vi "Data_get.vi"() -> ()   [LabVIEW 2009]
uses:
  <vilib>/Analysis/2dsp.llb/Real FFT.vi
  <vilib>/Analysis/NI_AALPro.lvlib
panel:
  in  "Auto":bool caption="Autosave"
  in  "FFT every#":u32=1 min=1 max=1000 step=1
  in  "#steps":u32=1 min=1 step=1
  in  "f step (MHz)":dbl=0.0003 min=0.00025 max=67.0 step=1e-06 format="%#.12f"
  in  "ps/point":T1(ring)
  in  "ns/div":T2(ring)
  out "Current sweep":u32=1 min=1 max=1000 step=1
  in  "Ext":string="ccd"
  out "f cur. (MHz)":string
  in  "Name":string="trace"
  in  "Folder":path
  in  "#Sweeps":u32=1 min=1 max=1000 step=1
  in  "Ampl. (dBm)":dbl min=-135.0 max=30.0 step=0.5 format="%#_8g"
  in  "f start (MHz)":dbl=0.0003 min=0.00025 max=67.0 step=1e-06 format="%#.12f"
  in  "Start":bool
  in  "Quit":bool
  in  "E8257D VISA Port":refnum<visa-resource-name>="GPIB0::1::INSTR"
  out "read time (ms)":u32
  out "#points":u32
  out "Busy":bool
  in  "Repetition rate (Hz)":ext=2.5
  in  "Chirp start (MHz)":ext=2.5
  in  "Filter up to (MHz)":ext=2.5
  in  "Amount of averagings":u32=10
  out "Data":dbl[](array[numeric])
  out "XY Graph 5":cluster{ext[], dbl[]}(graph)
  out "FFT (Im)":dbl[](array[numeric])
  out "FFT (Re)":dbl[](array[numeric])
  out "Final array":ext[][](array[numeric])
  out "size(s)":i32
  out "Oscilloscope Data":dbl[](array[numeric])
  in  "Channel Number":u16=1
  out "Oscilloscope graph":dbl[](graph)
  in  "Stop":bool
  in  "TDS VISA Port":refnum<visa-resource-name>="GPIB0::1::INSTR"
  # "TDS6000"
  # "E8257D"
  # "File Storage"
  # "Control"
  # "Spectrum data"
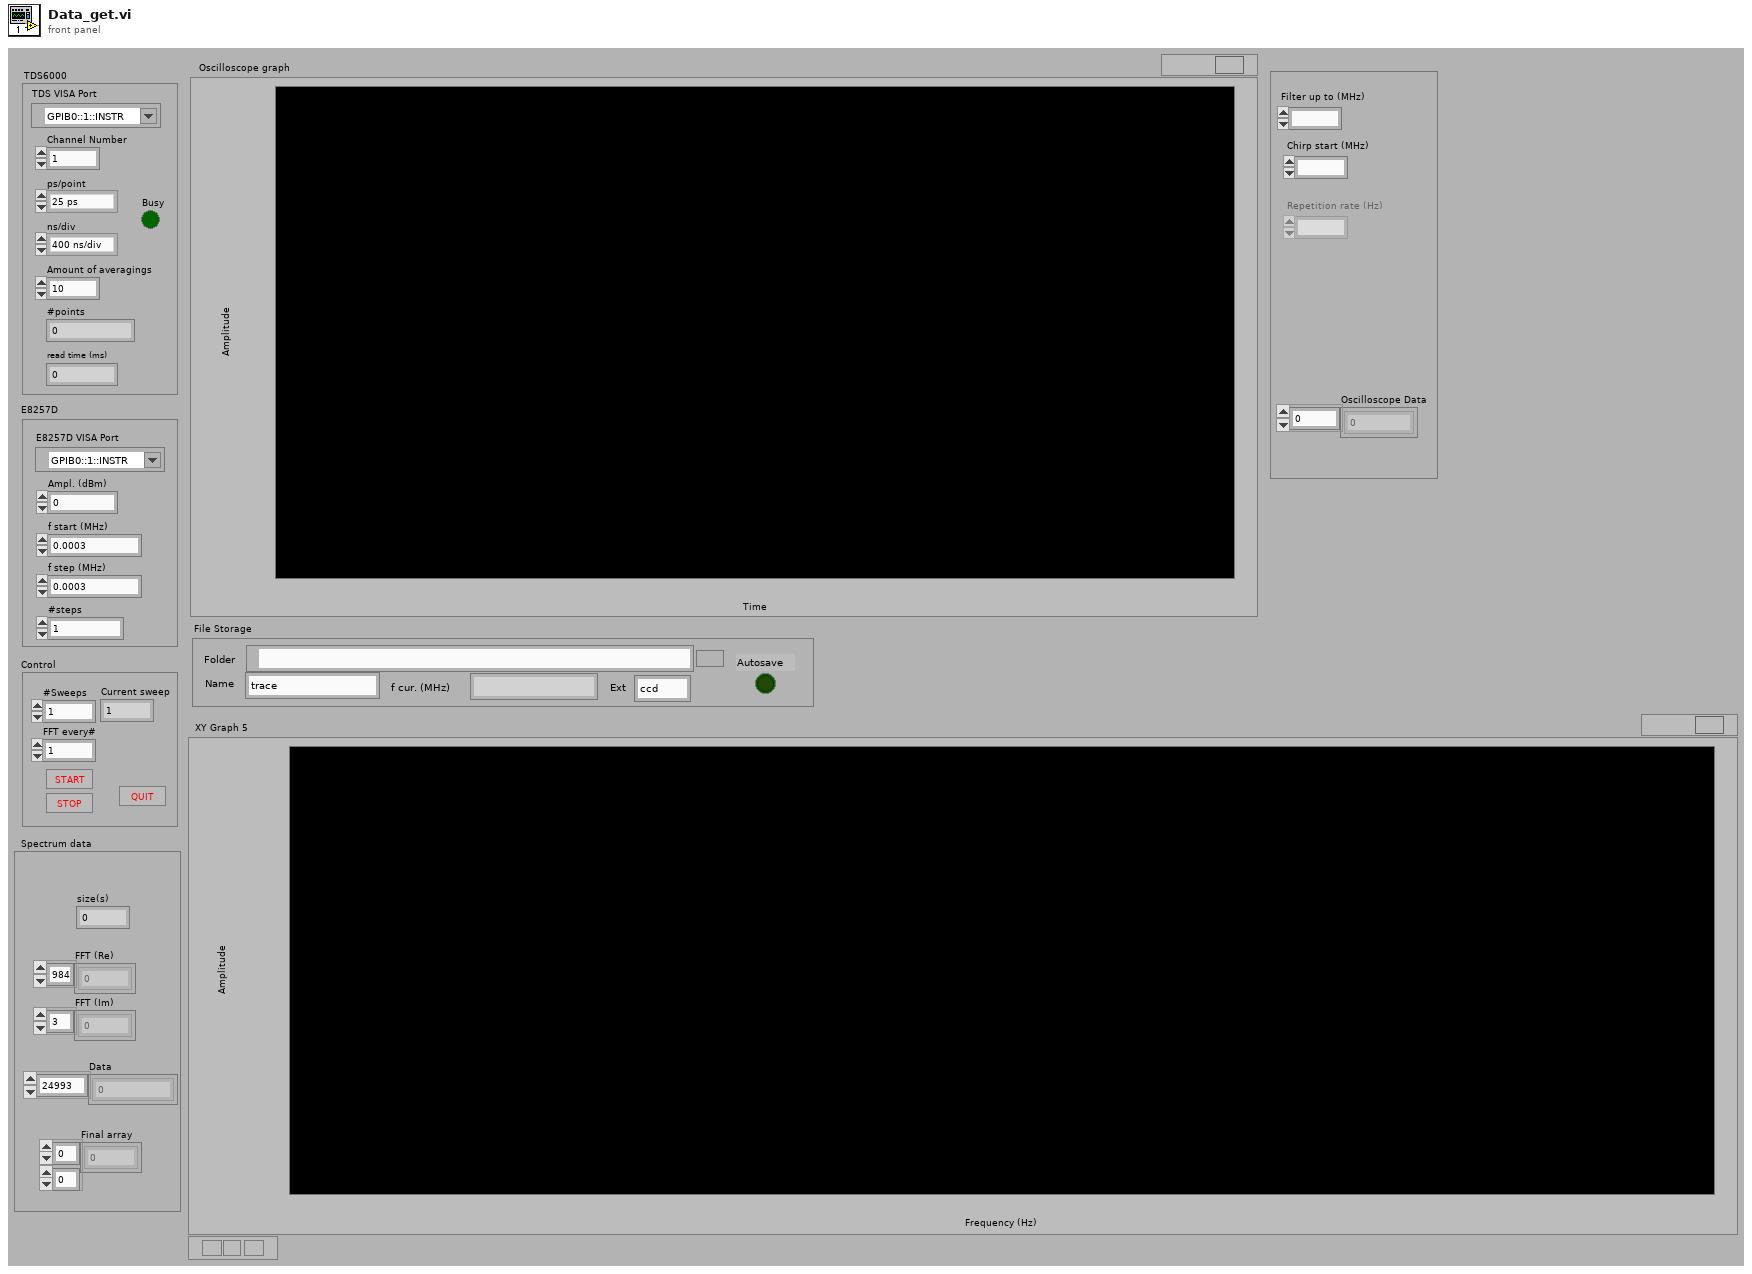
[diagram p1: front panel]
types:
  T1 = enum16{"25 ps", "50 ps", "100 ps", "200 ps", "400 ps", "800 ps", "2 ns"}
  T2 = enum16{"400 ns/div", "1 us/div", "2 us/div", "4 us/div", "10 us/div", "20 us/div"}
  T3 = enum16{"open", "replace", "create", "open or create", "replace or create", "replace or create with confirmation"}
  T4 = cluster{"Folder":path, "Name":string, "Ext":string}
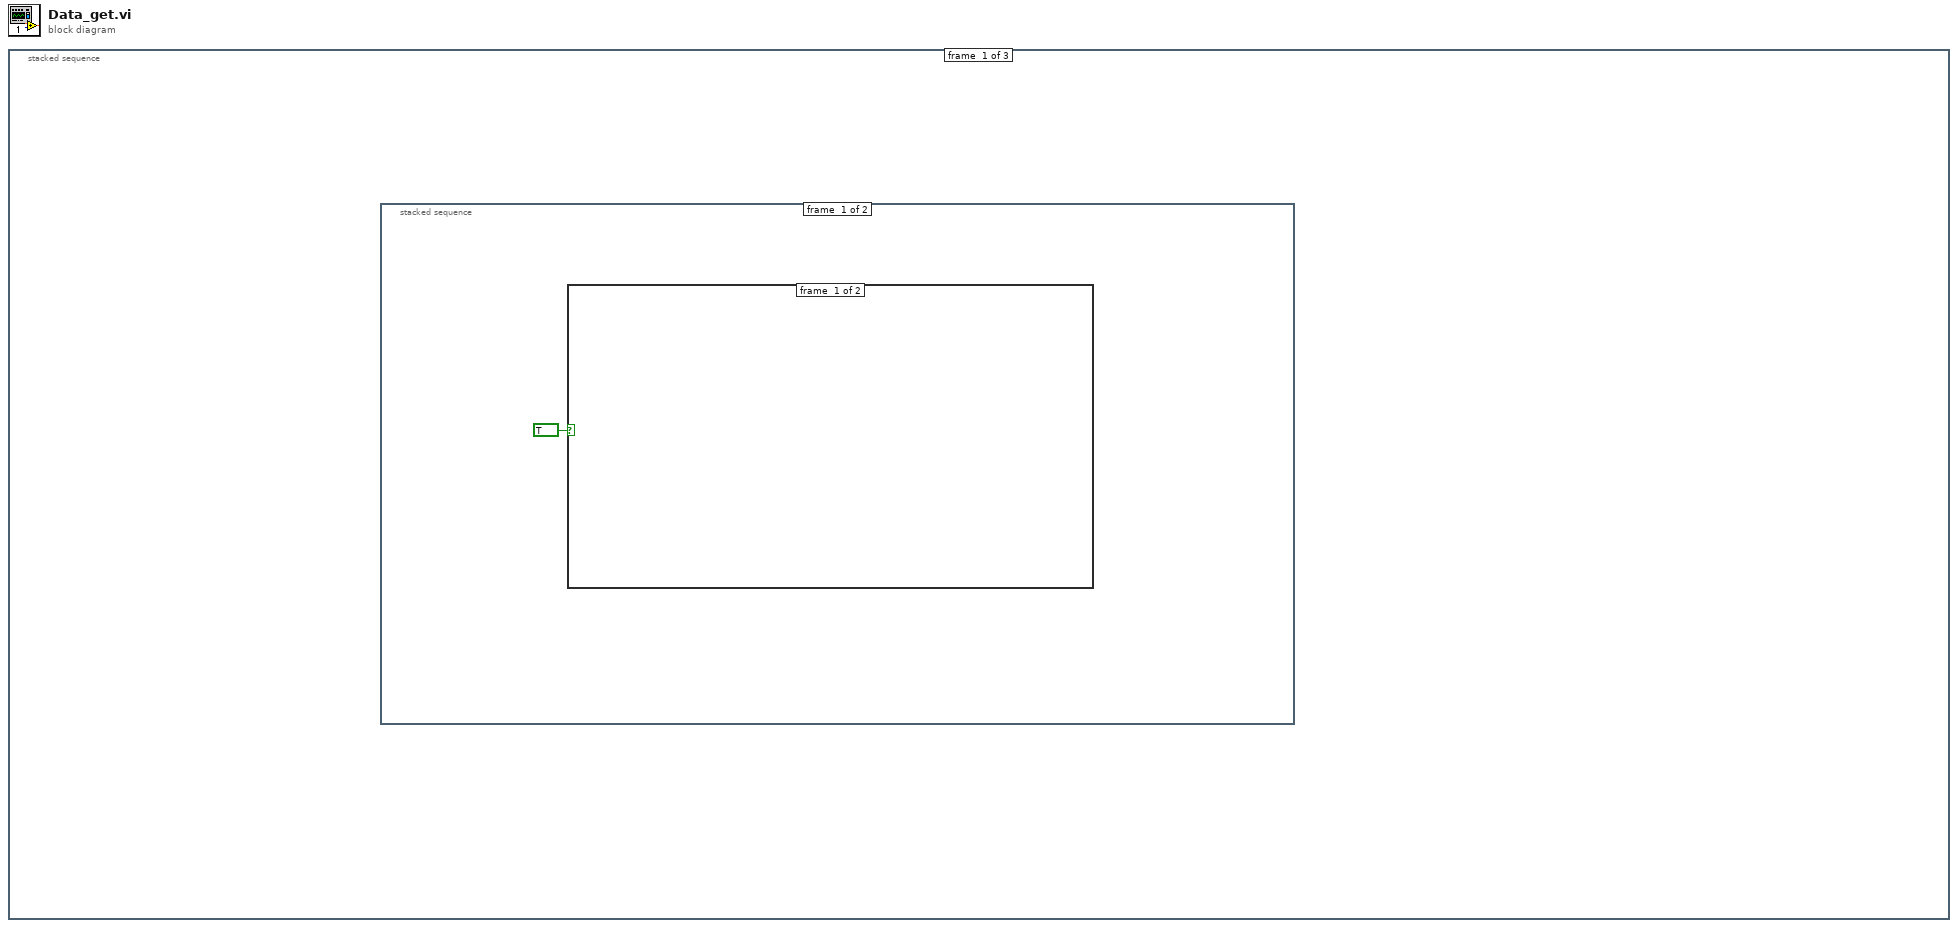
[diagram p0: block diagram]
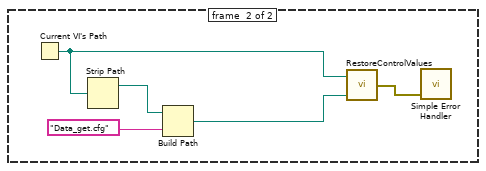
[diagram p2: hidden frame]
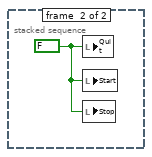
[diagram p3: hidden frame]
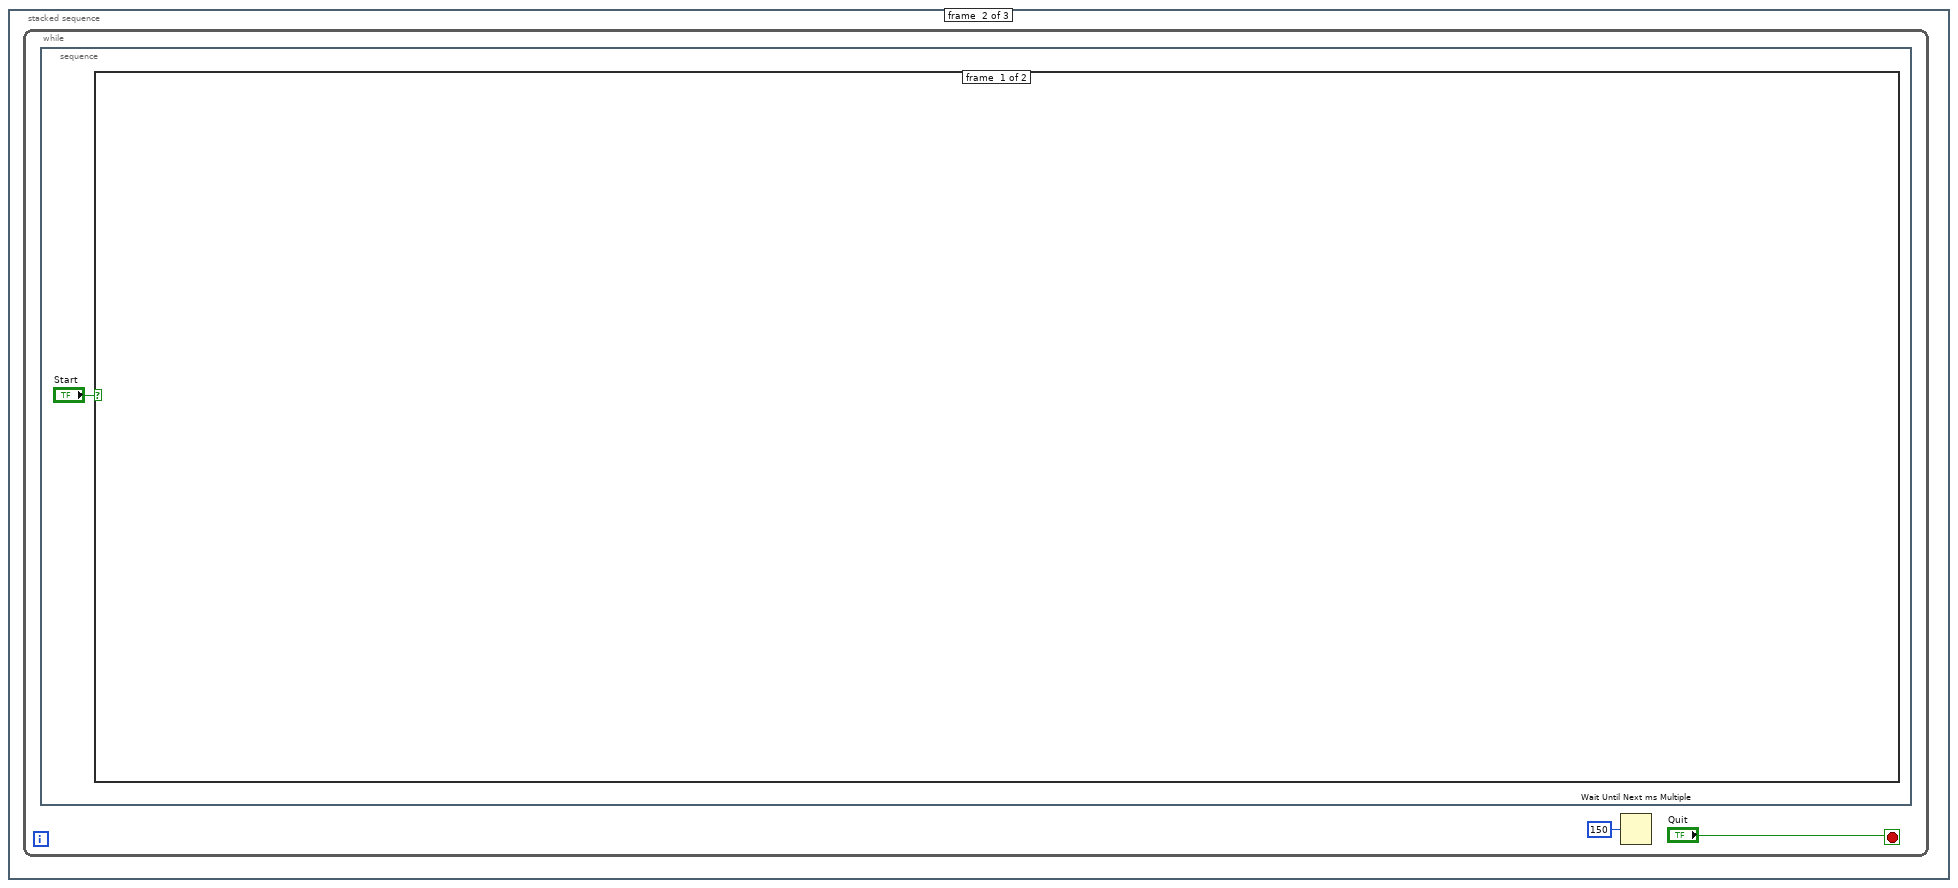
[diagram p4: hidden frame]
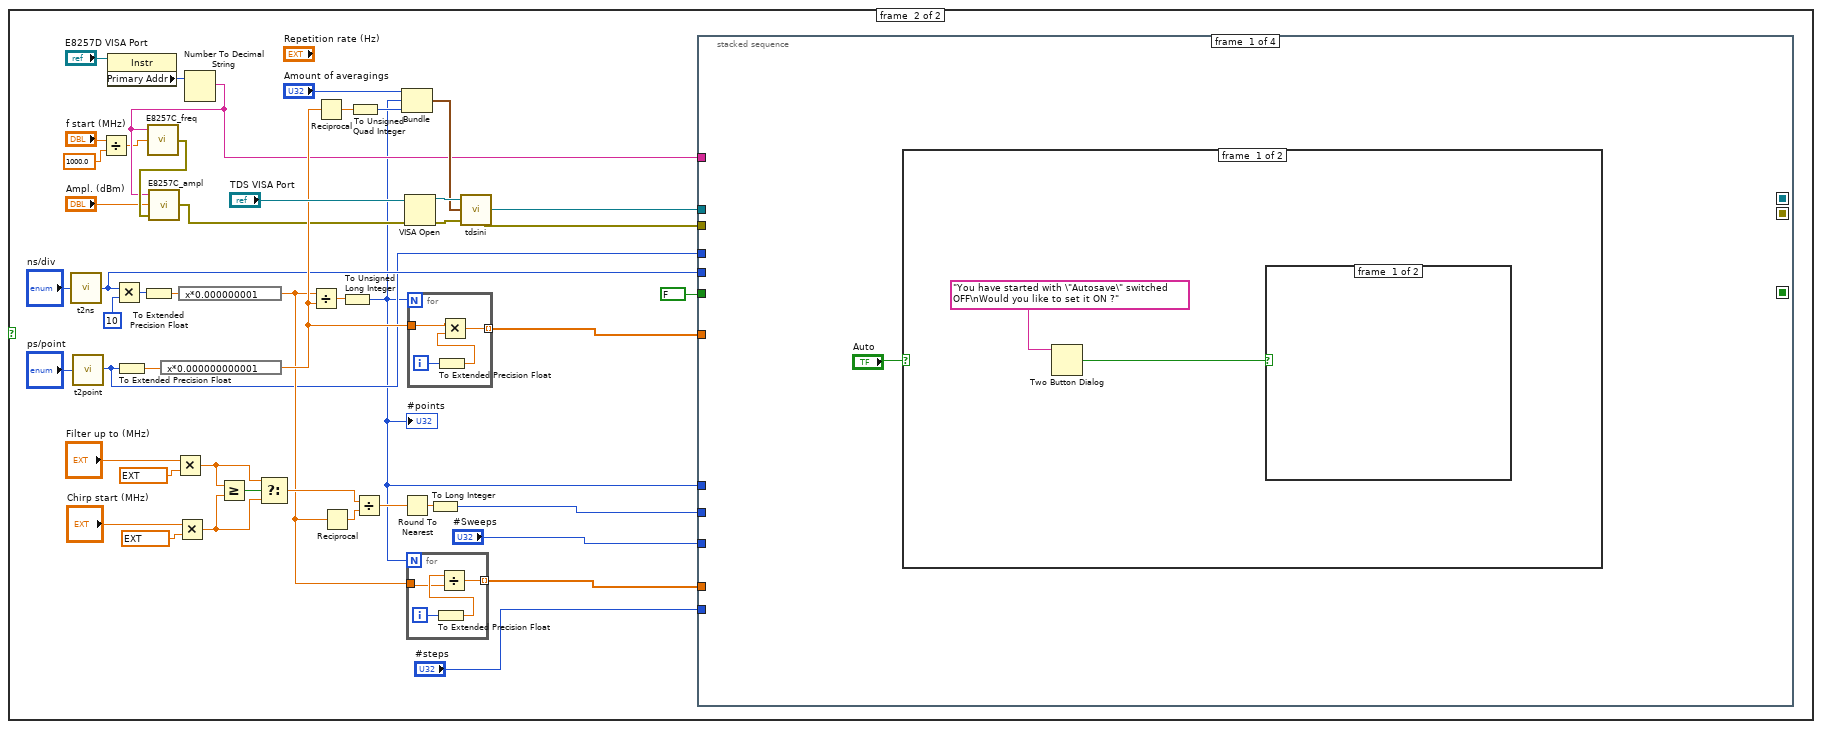
[diagram p5: hidden frame]
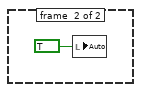
[diagram p6: hidden frame]
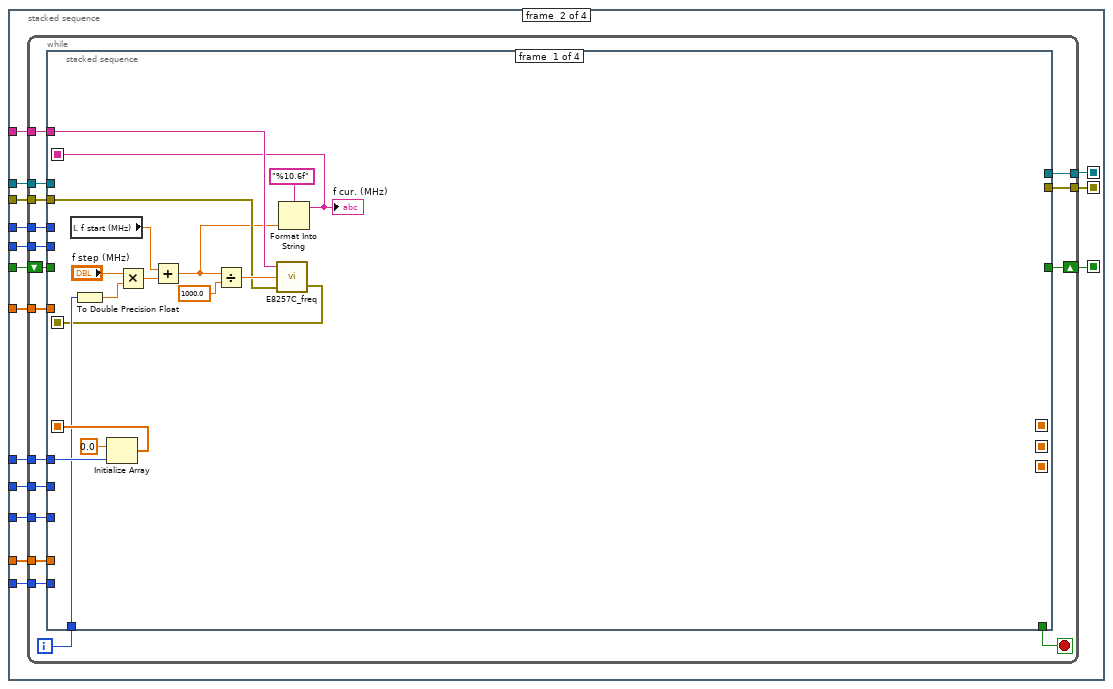
[diagram p8: hidden frame]
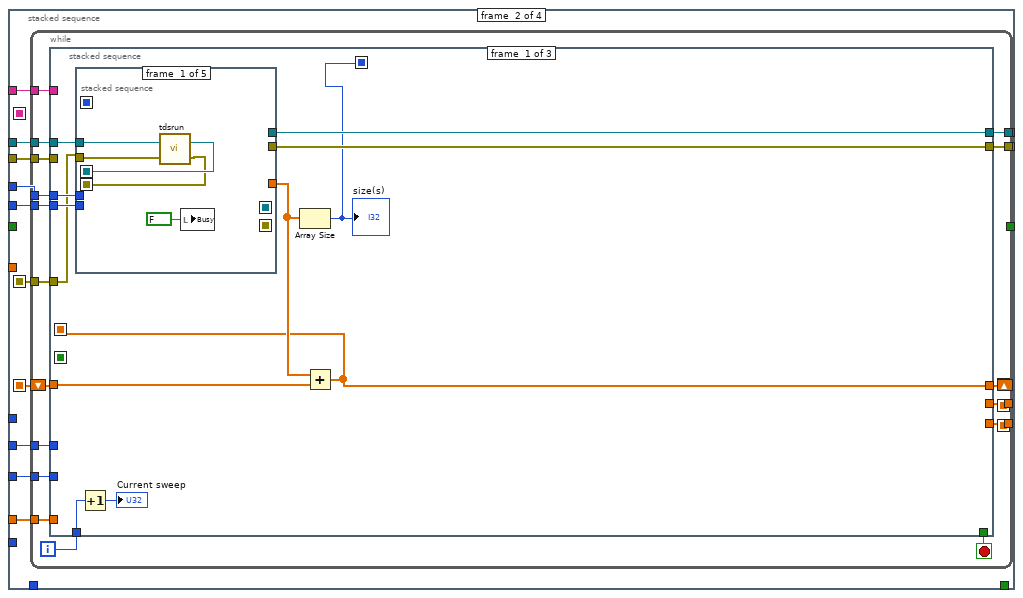
[diagram p9: hidden frame]
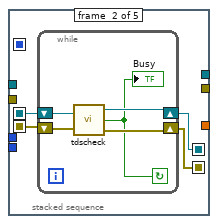
[diagram p10: hidden frame]
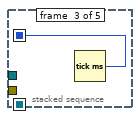
[diagram p11: hidden frame]
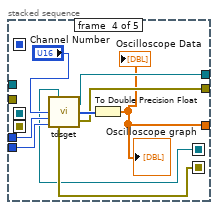
[diagram p12: hidden frame]
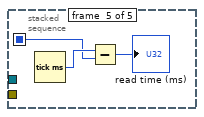
[diagram p13: hidden frame]
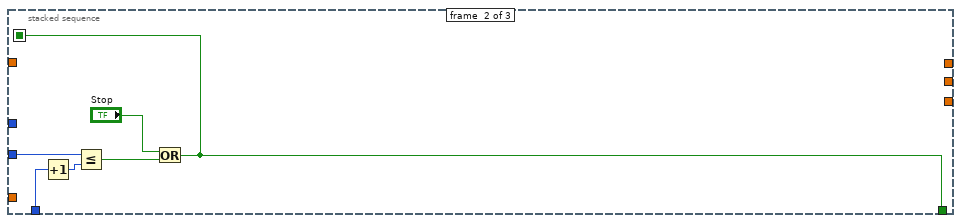
[diagram p14: hidden frame]
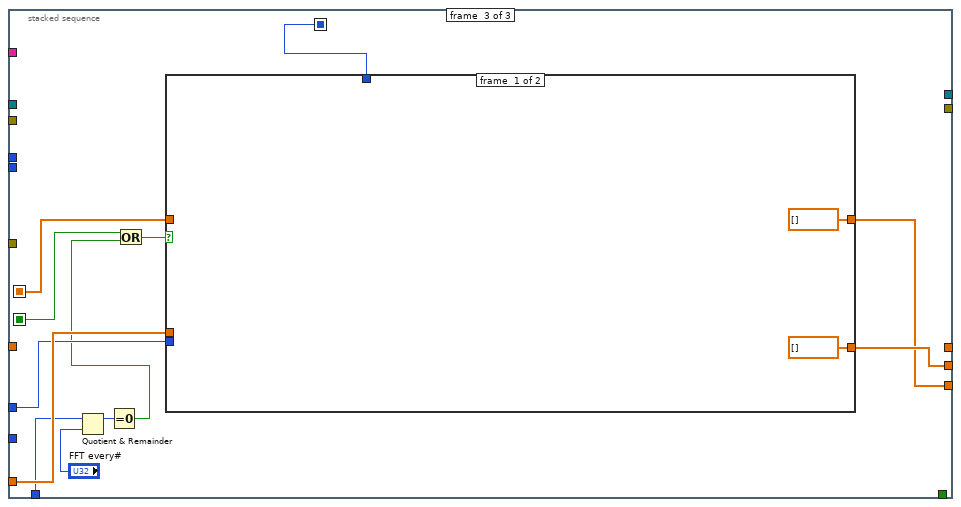
[diagram p15: hidden frame]
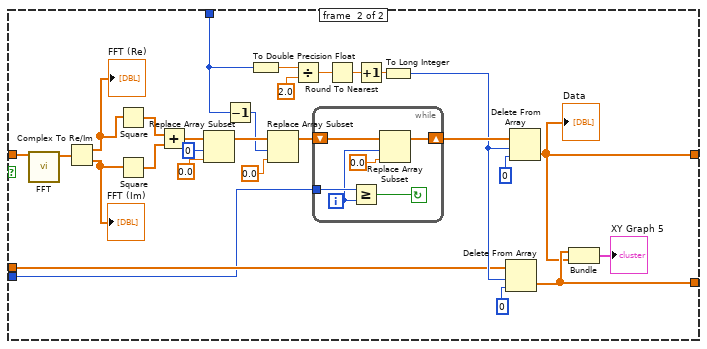
[diagram p16: hidden frame]
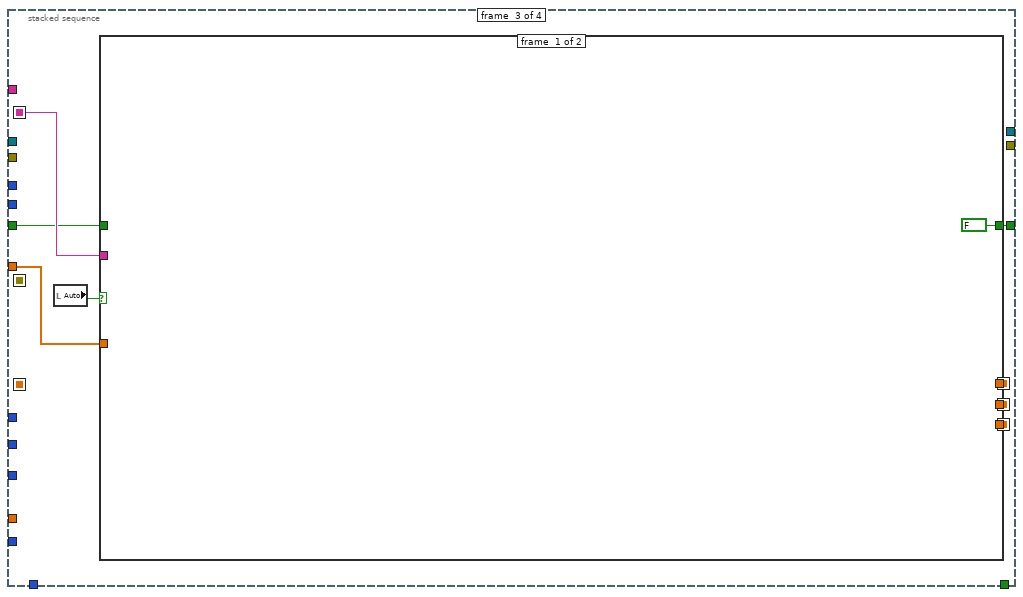
[diagram p17: hidden frame]
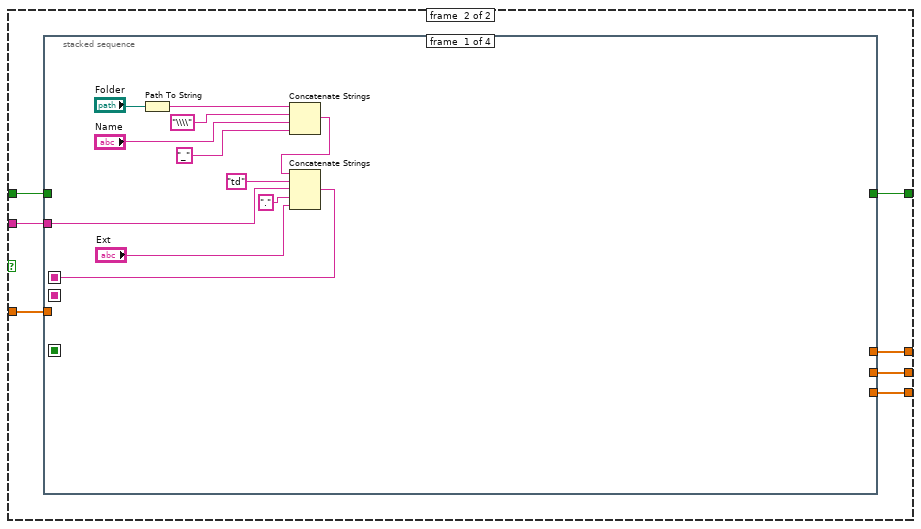
[diagram p18: hidden frame]
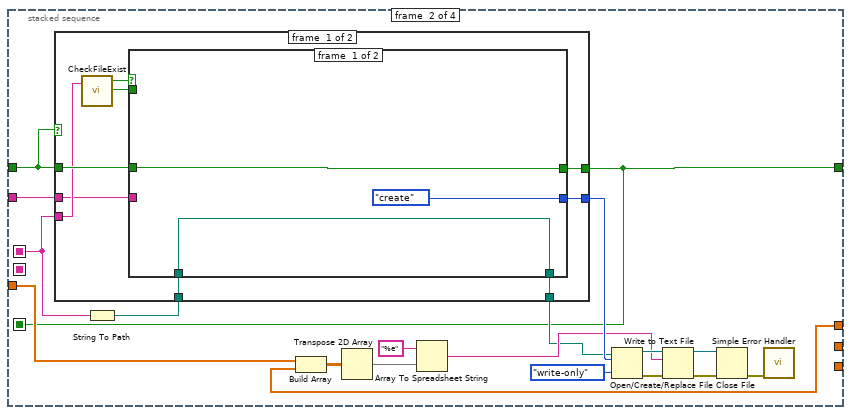
[diagram p19: hidden frame]
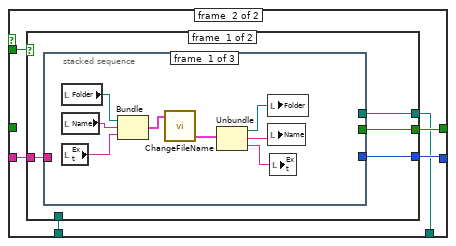
[diagram p20: hidden frame]
diagram:
  n1 = stacked-sequence {
    frame #0 {
      n2 = stacked-sequence {
        frame #0 {
          n3 = case shown="True" TRUE {
            frame #0 {
            }
            frame #1 {
              n4 = Current VI's Path() -> (path=w2:path)
              n5 = Strip Path(path=w2) -> (stripped path=w3:path)  [unwired: 1 out]
              n6 = Build Path(base path=w3, name or relative path="Data_get.cfg") -> (appended path=w5:path)
              n7 = call "RestoreControlValues.vi"("file path"=w5, "vi path"=w2) -> ("error out"=w4:errorcluster)
              n8 = call <vilib>:"Simple Error Handler.vi"("error in (no error)"=w4) -> ()  [unwired: 4 in, 5 out]
            }
          }
        }
        frame #1 {
          w7 = FALSE ("Quit")
          n9 = local write "Quit"(w7) -> ()
          n10 = local write "Start"(w7) -> ()
          n11 = local write "Stop"(w7) -> ()
        }
      }
    }
    frame #1 {
      n12 = while {
        stop <- "Quit" stop-if-true
        n13 = stacked-sequence {
          frame #0 {
            n14 = case shown="True" "Start" {
              frame #0 {
              }
              frame #1 {
                n15 = call "t2ns.vi"("t/div"="ns/div") -> ("ns/div"=w17:u32)
                n16 = call "t2point.vi"("t/point"="ps/point") -> ("ps/point"=w15:u32)
                n17 = Divide(x="f start (MHz)", y=1000.0) -> (x/y=w20:dbl)
                n18 = property class="Instr"(reference="E8257D VISA Port") -> ("Primary Addr"=w27:u16)  [unwired: 1 in, 2 out]
                n19 = Multiply(x=w17, y=u32 10) -> (x*y=w51:u32)
                n20 = To Extended Precision Float(1:w15) -> (0:w48:ext)
                n21 = To Extended Precision Float(1:w51) -> (0:w49:ext)
                n22 = expression code="x*0.000000000001"(w48) -> (w33:ext)
                n23 = Multiply(x="Filter up to (MHz)", y=ext 1000000.0) -> (x*y=w39:ext)
                n24 = Multiply(x="Chirp start (MHz)", y=ext 1000000.0) -> (x*y=w36:ext)
                n25 = expression code="x*0.000000001"(w49) -> (w29:ext)
                n26 = Number To Decimal String(number=w27) -> (decimal integer string=w24:string)  [unwired: 1 in]
                n27 = call "E8257C_freq.vi"("Frequency GHz"=w20, "GPIB address"=w24) -> ("error out"=w25:errorcluster)  [unwired: 1 in]
                n28 = call "E8257C_ampl.vi"("error in"=w25, "Amplitude dBm"="Ampl. (dBm)", "GPIB address"=w24) -> ("error out"=w23:errorcluster)
                n29 = Greater Or Equal?(x=w39, y=w36) -> (x >= y?=w47:bool)
                n30 = Select(t=w39, s=w47, f=w36) -> (s? t:f=w45:ext)
                n31 = Divide(x=w29, y=w33) -> (x/y=w50:ext)
                n32 = Reciprocal(x=w33) -> (1/x=w31:ext)
                n33 = Reciprocal(x=w29) -> (1/x=w46:ext)
                n34 = To Unsigned Long Integer(number=w50) -> (unsigned 32bit integer=w13:u32)
                "#points" <- w13
                n35 = To Unsigned Quad Integer(1:w31) -> (0:w32:u64)
                n36 = Divide(x=w45, y=w46) -> (x/y=w44:ext)
                n37 = Bundle("Amount of averagings"="Amount of averagings", w13, w32) -> (w34:cluster{"Amount of averagings ":u32, u32, u64})  [unwired: 1 in]
                n38 = Round To Nearest(number=w44) -> (nearest integer value=w43:ext)
                n39 = VISA Open(error in (no error)=w23, VISA resource name="TDS VISA Port") -> (VISA resource name=w54:refnum<visa-resource-name>, error out=w55:errorcluster)  [unwired: 3 in]
                n40 = for {
                  N: w13 -> [_]
                  tunnel: w29 -> [w409]
                  tunnel: [w411] -> w30 mode=indexing
                  i -> [w412]
                  n41 = To Extended Precision Float(1:w412) -> (0:w410:ext)
                  n42 = Divide(x=w410, y=w409) -> (x/y=w411:ext)
                }
                n43 = for {
                  N: w13 -> [_]
                  tunnel: w33 -> [w414]
                  tunnel: [w413] -> w18 mode=indexing
                  i -> [w416]
                  n44 = To Extended Precision Float(1:w416) -> (0:w415:ext)
                  n45 = Multiply(x=w414, y=w415) -> (x*y=w413:ext)
                }
                n46 = To Long Integer(number=w43) -> (32bit integer=w42:i32)
                n47 = call "tdsini.vi"("Error In (No Error)"=w55, "Acq_par"=w34, "VISA Port In"=w54) -> ("Error Out"=w56:errorcluster, "VISA Port Out"=w57:refnum<visa-resource-name>)
                n48 = stacked-sequence {
                  seq-local: [_ w68 _ _] -> [_ _ w370 _]
                  seq-local: [_ w67 _ _] -> [_ _ w369 _]
                  seq-local: [_ w62 _ _] -> [_ _ _ w371]
                  tunnel: w57 -> [_ w76 _ _]
                  tunnel: w56 -> [_ w75 _ _]
                  tunnel: w15 -> [_ w74 _ _]
                  tunnel: w17 -> [_ w73 _ _]
                  tunnel: w42 -> [_ w72 _ _]
                  tunnel: w30 -> [_ w71 _ _]
                  tunnel: w24 -> [_ w70 w367 _]
                  tunnel: "#Sweeps" -> [_ w69 _ _]
                  tunnel: w18 -> [_ w64 _ _]
                  tunnel: w13 -> [_ w66 _ _]
                  tunnel: "#steps" -> [_ w65 _ _]
                  tunnel: FALSE -> [_ w63 _ _]
                  frame #0 {
                    n49 = case shown="False" "Auto" {
                      frame #0 {
                        n50 = Two Button Dialog(message="You have started with \"Autosave\" switched OFF\nWould you like to set it ON ?") -> (T button?=w59:bool)  [unwired: 2 in]
                        n51 = case shown="True" w59 {
                          frame #0 {
                          }
                          frame #1 {
                            n52 = local write "Auto"(TRUE) -> ()
                          }
                        }
                      }
                      frame #1 {
                      }
                    }
                  }
                  frame #1 {
                    n53 = while {
                      tunnel: w76 -> [w93]
                      tunnel: w75 -> [w92]
                      tunnel: w74 -> [w91]
                      tunnel: w73 -> [w90]
                      tunnel: w72 -> [w89]
                      tunnel: w71 -> [w88]
                      tunnel: w70 -> [w87]
                      tunnel: w69 -> [w86]
                      tunnel: [w85] -> w68
                      tunnel: [w84] -> w67
                      tunnel: w66 -> [w83]
                      tunnel: w65 -> [w81]
                      tunnel: w64 -> [w79]
                      shift-right: [w77] -> w62
                      shift-left: w63 -> [w78]
                      i -> [w82]
                      stop <- w80 stop-if-true
                      n54 = stacked-sequence {
                        seq-local: [w108 _ _ _] -> [_ w114 _ _]
                        seq-local: [w97 _ _ _] -> [_ w113 _ _]
                        seq-local: [_ w112 _ _] -> [_ _ w241 _]
                        seq-local: [_ w111 _ _] -> [_ _ w240 _]
                        seq-local: [_ w110 _ _] -> [_ _ w239 _]
                        seq-local: [w94 _ _ _] -> [_ _ w238 _]
                        tunnel: w93 -> [_ w124 _ _]
                        tunnel: w92 -> [w98 w123 _ _]
                        tunnel: w91 -> [_ w122 _ _]
                        tunnel: w90 -> [_ w121 _ _]
                        tunnel: w89 -> [_ w120 _ _]
                        tunnel: w88 -> [_ w119 _ _]
                        tunnel: w87 -> [w99 w118 _ _]
                        tunnel: w86 -> [_ w117 _ _]
                        tunnel: [_ w116 _ _] -> w85
                        tunnel: [_ w115 _ _] -> w84
                        tunnel: w83 -> [w107 _ _ _]
                        tunnel: w82 -> [w102 _ _ w363]
                        tunnel: w81 -> [_ _ _ w362]
                        tunnel: [_ _ _ w361] -> w80
                        tunnel: w79 -> [_ _ w242 _]
                        tunnel: w78 -> [_ _ w236 _]
                        tunnel: [_ _ w235 _] -> w77
                        frame #0 {
                          n55 = local read "f start (MHz)"() -> (w100:dbl)
                          n56 = To Double Precision Float(number=w102) -> (double precision float=w103:dbl)
                          n57 = Initialize Array(0.0 ("element"), w107) -> (w108:dbl[])
                          n58 = Multiply(x="f step (MHz)", y=w103) -> (x*y=w101:dbl)
                          n59 = Add(x=w100, y=w101) -> (x+y=w96:dbl)
                          n60 = Divide(x=w96, y=1000.0) -> (x/y=w106:dbl)
                          n61 = call "E8257C_freq.vi"("error in"=w98, "Frequency GHz"=w106, "GPIB address"=w99) -> ("error out"=w97:errorcluster)
                          n62 = Format Into String(format string="%10.6f", w96) -> (resulting string=w94:string)  [unwired: 2 in, 1 out]
                          "f cur. (MHz)" <- w94
                        }
                        frame #1 {
                          n63 = while {
                            tunnel: [w138] -> w115
                            tunnel: [w139] -> w116
                            tunnel: w123 -> [w140]
                            tunnel: w124 -> [w141]
                            tunnel: w122 -> [w137]
                            tunnel: w121 -> [w136]
                            tunnel: w119 -> [w134]
                            tunnel: w120 -> [w135]
                            tunnel: w118 -> [w131]
                            tunnel: w117 -> [w130]
                            shift-right: [w128] -> w112
                            shift-left: w114 -> [w129]
                            tunnel: [w127] -> w111
                            tunnel: w113 -> [w126]
                            tunnel: [w125] -> w110
                            i -> [w133]
                            stop <- w132 stop-if-true
                            n64 = stacked-sequence {
                              seq-local: [w142 _ _] -> [_ _ w198]
                              seq-local: [w143 _ _] -> [_ _ w197]
                              seq-local: [_ w181 _] -> [_ _ w188]
                              tunnel: w141 -> [w153 _ _]
                              tunnel: w140 -> [_ _ _]
                              tunnel: [w152 _ _] -> w139
                              tunnel: [w151 _ _] -> w138
                              tunnel: w137 -> [w150 _ _]
                              tunnel: w136 -> [w149 _ _]
                              tunnel: w135 -> [_ _ w195]
                              tunnel: w134 -> [_ _ w196]
                              tunnel: w133 -> [w146 w186 w192]
                              tunnel: [_ w181 _] -> w132
                              tunnel: w131 -> [_ _ _]
                              tunnel: w130 -> [_ w183 _]
                              tunnel: w129 -> [w148 _ _]
                              tunnel: [w143 _ _] -> w128
                              tunnel: [_ _ w194] -> w127
                              tunnel: w126 -> [w145 _ _]
                              tunnel: [_ _ w193] -> w125
                              frame #0 {
                                n65 = stacked-sequence {
                                seq-local: [w156 _ _ _ _] -> [_ w162 _ _ _]
                                seq-local: [w155 _ _ _ _] -> [_ w161 _ _ _]
                                seq-local: [_ w159 _ _ _] -> [_ _ _ w170 _]
                                seq-local: [_ w160 _ _ _] -> [_ _ _ w169 _]
                                seq-local: [_ _ w168 _ _] -> [_ _ _ _ w179]
                                tunnel: w153 -> [w157 _ _ _ _]
                                tunnel: w145 -> [w158 _ _ _ _]
                                tunnel: [_ _ _ w176 _] -> w152
                                tunnel: [_ _ _ w175 _] -> w151
                                tunnel: w150 -> [_ _ _ w173 _]
                                tunnel: w149 -> [_ _ _ w172 _]
                                tunnel: [_ _ _ w171 _] -> w144
                                frame #0 {
                                n66 = call "tdsrun.vi"("Error In (No Error)"=w158, "VISA Port In"=w157) -> ("Error Out"=w155:errorcluster, "VISA Port Out"=w156:refnum<visa-resource-name>)
                                n67 = local write "Busy"(FALSE ("Busy")) -> ()
                                }
                                frame #1 {
                                n68 = while {
                                shift-right: [w165] -> w160
                                shift-left: w162 -> [w166]
                                shift-right: [w164] -> w159
                                shift-left: w161 -> [w167]
                                stop <- w163 continue-if-true
                                n69 = call "tdscheck.vi"("VISA Port In"=w166, "Error In (No Error)"=w167) -> ("VISA Port Out"=w165:refnum<visa-resource-name>, "busy"=w163:bool, "Error Out"=w164:errorcluster)
                                "Busy" <- w163
                                }
                                }
                                frame #2 {
                                n70 = Tick Count (ms)() -> (millisecond timer value=w168:u32)
                                }
                                frame #3 {
                                n71 = call "tdsget.vi"("VISA Port In"=w169, "Channel Number"="Channel Number", "ps/point"=w173, "ns/div"=w172, "Error In (No Error)"=w170) -> ("VISA Port Out"=w176:refnum<visa-resource-name>, "TDS Data"=w177:u16[], "Error Out"=w175:errorcluster)  [unwired: 8 in]
                                n72 = To Double Precision Float(number=w177) -> (double precision float=w171:dbl[])
                                "Oscilloscope graph" <- w171
                                "Oscilloscope Data" <- w171
                                }
                                frame #4 {
                                n73 = Tick Count (ms)() -> (millisecond timer value=w180:u32)
                                n74 = Subtract(x=w180, y=w179) -> (x-y=→"read time (ms)":u32)
                                }
                                }
                                n75 = Increment(x=w146) -> (x+1=→"Current sweep":i32)
                                n76 = Array Size(array=w144) -> (size(s)=w142:i32)
                                "size(s)" <- w142
                                n77 = Add(x=w144, y=w148) -> (x+y=w143:dbl[])
                              }
                              frame #1 {
                                n78 = Increment(x=w186) -> (x+1=w182:i32)
                                n79 = Less Or Equal?(x=w183, y=w182) -> (x <= y?=w185:bool)
                                n80 = Or(x="Stop", y=w185) -> (x .or. y?=w181:bool)
                              }
                              frame #2 {
                                n81 = Quotient & Remainder(x=w192, y="FFT every#") -> (x-y*floor(x/y)=w190:u32)  [unwired: 1 out]
                                n82 = Equal To 0?(x=w190) -> (x = 0?=w187:bool)
                                n83 = Or(x=w188, y=w187) -> (x .or. y?=w189:bool)
                                n84 = case shown="True" w189 {
                                tunnel: w198 -> [_ w206]
                                tunnel: w197 -> [_ w205]
                                tunnel: w196 -> [_ w204]
                                tunnel: w195 -> [_ w203]
                                tunnel: [ext[] [] w202] -> w194
                                tunnel: [dbl[] [] w201] -> w193
                                frame #0 {
                                }
                                frame #1 {
                                n85 = call-poly <vilib>:"FFT.vi"("X"=w205) -> ("FFT {X}"=w228:cdb[])  [unwired: 9 in, 1 out]
                                n86 = Complex To Re/Im(x + iy=w228) -> (x=w227:dbl[], y=w226:dbl[])
                                "FFT (Re)" <- w227
                                "FFT (Im)" <- w226
                                n87 = Square(x=w227) -> (x^2=w225:dbl[])
                                n88 = Square(x=w226) -> (x^2=w224:dbl[])
                                n89 = Add(x=w225, y=w224) -> (x+y=w220:dbl[])
                                n90 = Replace Array Subset(array=w220, new element=0.0 ("new element/subarray"), index=0) -> (w219:dbl[])
                                n91 = Decrement(x=w206) -> (x-1=w218:i32)
                                n92 = To Double Precision Float(number=w206) -> (double precision float=w214:dbl)
                                n93 = Replace Array Subset(array=w219, new element=0.0 ("new element/subarray"), index=w218) -> (w216:dbl[])
                                n94 = Divide(x=w214, y=2.0) -> (x/y=w212:dbl)
                                n95 = while {
                                tunnel: w203 -> [w233]
                                shift-right: [w231] -> w215
                                shift-left: w216 -> [w232]
                                i -> [w230]
                                stop <- w234 continue-if-true
                                n96 = Greater Or Equal?(x=w233, y=w230) -> (x >= y?=w234:bool)
                                n97 = Replace Array Subset(array=w232, new element=0.0 ("new element/subarray"), index=w230) -> (w231:dbl[])
                                }
                                n98 = Round To Nearest(number=w212) -> (nearest integer value=w211:dbl)
                                n99 = Increment(x=w211) -> (x+1=w210:dbl)
                                n100 = To Long Integer(number=w210) -> (32bit integer=w207:i32)
                                n101 = Delete From Array(array=w204, length=w207, index=0) -> (deleted portion=w202:ext[])  [unwired: 1 out]
                                n102 = Delete From Array(array=w215, length=w207, index=0) -> (deleted portion=w201:dbl[])  [unwired: 1 out]
                                "Data" <- w201
                                n103 = Bundle(w202, w201) -> (→"XY Graph 5":cluster{ext[], dbl[]})  [unwired: 1 in]
                                }
                                }
                              }
                            }
                          }
                        }
                        frame #2 {
                          n104 = local read "Auto"() -> (w237:bool)
                          n105 = case shown="True" w237 {
                            tunnel: w242 -> [_ w250]
                            tunnel: w241 -> [_ w249]
                            tunnel: w240 -> [_ w248]
                            tunnel: w239 -> [_ w247]
                            tunnel: w238 -> [_ w246]
                            tunnel: w236 -> [_ w245]
                            tunnel: [FALSE w244] -> w235
                            frame #0 {
                            }
                            frame #1 {
                              n106 = stacked-sequence {
                                seq-local: [w251 _ _ _] -> [_ w276 _ _]
                                seq-local: [_ _ w331 _] -> [_ _ _ w352]
                                seq-local: [_ w263 _ _] -> [_ _ _ w343]
                                tunnel: w250 -> [_ w278 _ _]
                                tunnel: w249 -> [_ w265 _ _]
                                tunnel: w248 -> [_ _ _ w355]
                                tunnel: w247 -> [_ _ _ w354]
                                tunnel: w246 -> [w253 w264 w333 _]
                                tunnel: w245 -> [_ w268 _ _]
                                tunnel: [_ w263 _ _] -> w244
                                frame #0 {
                                n107 = Path To String(path="Folder") -> (string=w261:string)
                                n108 = Concatenate Strings(w261, "\\\\" ("string"), "Name", "_") -> (w252:string)
                                n109 = Concatenate Strings(w252, "td", w253, ".", "Ext") -> (w251:string)
                                }
                                frame #1 {
                                n110 = String To Path(string=w276) -> (path=w267:path)
                                n111 = case shown="False" w268 {
                                tunnel: w276 -> [w282 _]
                                tunnel: [w287 w329] -> w263
                                tunnel: [w285 T3."replace or create" ("operation (0:open)")] -> w270
                                tunnel: w268 -> [w286 w329]
                                tunnel: w267 -> [w284 w328]
                                tunnel: [w283 w328] -> w266
                                tunnel: w264 -> [w281 _]
                                frame #0 {
                                n112 = call "CheckFileExist.vi"("Path"=w282) -> ("Exist"=w289:bool, "Overwrite"=w288:bool)  [unwired: 1 in, 1 out]
                                n113 = case shown="True" w289 {
                                tunnel: w288 -> [_ w298]
                                tunnel: [w292 w296] -> w287
                                tunnel: w286 -> [w292 _]
                                tunnel: [T3."create" ("operation (0:open)") w297] -> w285
                                tunnel: w284 -> [w290 w295]
                                tunnel: [w290 w294] -> w283
                                tunnel: w281 -> [_ w293]
                                frame #0 {
                                }
                                frame #1 {
                                n114 = case shown="True" w298 {
                                tunnel: [w301 T3."replace or create" ("operation (0:open)")] -> w297
                                tunnel: [w302 TRUE] -> w296
                                tunnel: w295 -> [_ w325]
                                tunnel: [w299 w325] -> w294
                                tunnel: w293 -> [w300 _]
                                frame #0 {
                                n115 = stacked-sequence {
                                tunnel: [_ _ FALSE] -> w302
                                tunnel: [_ _ T3."create" ("operation (0:open)")] -> w301
                                tunnel: w300 -> [_ w314 _]
                                tunnel: [_ w311 _] -> w299
                                frame #0 {
                                n116 = local read "Folder"() -> (w310:path)
                                n117 = local read "Name"() -> (w309:string)
                                n118 = local read "Ext"() -> (w308:string)
                                n119 = Bundle("Folder"=w310, "Name"=w309, "Ext"=w308) -> (w307:T4)  [unwired: 1 in]
                                n120 = call "ChangeFileName.vi"("input par"=w307) -> ("output par"=w306:T4)  [unwired: 1 out]
                                n121 = Unbundle(w306) -> ("Folder"=w305:path, "Name"=w304:string, "Ext"=w303:string)
                                n122 = local write "Folder"(w305) -> ()
                                n123 = local write "Name"(w304) -> ()
                                n124 = local write "Ext"(w303) -> ()
                                }
                                frame #1 {
                                n125 = local read "Folder"() -> (w319:path)
                                n126 = local read "Name"() -> (w318:string)
                                n127 = local read "Ext"() -> (w313:string)
                                n128 = Path To String(path=w319) -> (string=w322:string)
                                n129 = Concatenate Strings(w322, "\\\\" ("string"), w318, "_") -> (w315:string)
                                n130 = Concatenate Strings(w315, "td", w314, ".", w313) -> (w312:string)
                                n131 = String To Path(string=w312) -> (path=w311:path)
                                }
                                frame #2 {
                                }
                                }
                                }
                                frame #1 {
                                }
                                }
                                }
                                }
                                }
                                frame #1 {
                                }
                                }
                                n132 = Build Array(w278, w265) -> (w280:ext[][])
                                n133 = Transpose 2D Array(2D array=w280) -> (transposed array=w277:ext[][])
                                n134 = Array To Spreadsheet String(array=w277, 3:"%e") -> (spreadsheet string=w269:string)  [unwired: 1 in]
                                n135 = Open/Create/Replace File(file path (use dialog)=w266, operation (0:open)=w270, access (0:read/write)=enum16{"read/write", "read-only", "write-only"}."write-only") -> (refnum out=w272:refnum<file>, error out=w275:errorcluster)  [unwired: 3 in, 1 out]
                                n136 = Write to Text File(file (use dialog)=w272, text=w269, error in=w275) -> (refnum out=w273:refnum<file>, error out=w274:errorcluster)  [unwired: 1 in, 1 out]
                                n137 = Close File(refnum=w273, error in=w274) -> (error out=w262:errorcluster)  [unwired: 1 out]
                                n138 = call <vilib>:"Simple Error Handler.vi"("error in (no error)"=w262) -> ()  [unwired: 4 in, 5 out]
                                }
                                frame #2 {
                                n139 = local read "Folder"() -> (w335:path)
                                n140 = local read "Name"() -> (w334:string)
                                n141 = local read "Ext"() -> (w332:string)
                                n142 = Path To String(path=w335) -> (string=w341:string)
                                n143 = Concatenate Strings(w341, "\\\\" ("string"), w334, "_") -> (w336:string)
                                n144 = Concatenate Strings(w336, "sd", w333, ".", w332) -> (w331:string)
                                }
                                frame #3 {
                                n145 = To Extended Precision Float(1:w354) -> (0:w356:ext[])
                                n146 = String To Path(string=w352) -> (path=w345:path)
                                n147 = case shown="True" w343 {
                                tunnel: [T3."replace or create with confirmation" ("operation (0:open)") T3."replace or create" ("operation (0:open)")] -> w344
                                frame #0 {
                                }
                                frame #1 {
                                }
                                }
                                n148 = Build Array(w355, w356) -> (w353:ext[][])
                                n149 = Transpose 2D Array(2D array=w353) -> (transposed array=w357:ext[][])
                                "Final array" <- w357
                                n150 = Array To Spreadsheet String(array=w357, 3:"%e") -> (spreadsheet string=w346:string)  [unwired: 1 in]
                                n151 = Open/Create/Replace File(file path (use dialog)=w345, operation (0:open)=w344, access (0:read/write)=enum16{"read/write", "read-only", "write-only"}."write-only") -> (refnum out=w348:refnum<file>, error out=w351:errorcluster)  [unwired: 3 in, 1 out]
                                n152 = Write to Text File(file (use dialog)=w348, text=w346, error in=w351) -> (refnum out=w349:refnum<file>, error out=w350:errorcluster)  [unwired: 1 in, 1 out]
                                n153 = Close File(refnum=w349, error in=w350) -> (error out=w342:errorcluster)  [unwired: 1 out]
                                n154 = call <vilib>:"Simple Error Handler.vi"("error in (no error)"=w342) -> ()  [unwired: 4 in, 5 out]
                                }
                              }
                            }
                          }
                        }
                        frame #3 {
                          n155 = Increment(x=w363) -> (x+1=w365:i32)
                          n156 = Less Or Equal?(x=w362, y=w365) -> (x <= y?=w366:bool)
                          n157 = local read "Stop"() -> (w364:bool)
                          n158 = Or(x=w364, y=w366) -> (x .or. y?=w361:bool)
                        }
                      }
                    }
                  }
                  frame #2 {
                    n159 = call "E8257C_local.vi"("GPIB address"=w367) -> ("error out"=w368:errorcluster)  [unwired: 1 in]
                    n160 = call <vilib>:"Simple Error Handler.vi"("error in (no error)"=w368) -> ()  [unwired: 4 in, 5 out]
                    n161 = VISA Close(VISA resource name=w370, error in (no error)=w369) -> ()  [unwired: 1 out]
                  }
                  frame #3 {
                    n162 = local read "Auto"() -> (w372:bool)
                    n163 = case shown="True" w372 {
                      tunnel: w371 -> [_ w375]
                      frame #0 {
                      }
                      frame #1 {
                        n164 = local read "Channel Number"() -> (w405:u16)
                        n165 = local read "ps/point"() -> (w404:T1)
                        n166 = local read "ns/div"() -> (w403:T2)
                        n167 = local read "Amount of averagings"() -> (w402:u32)
                        n168 = local read "#Sweeps"() -> (w401:u32)
                        n169 = local read "Filter up to (MHz)"() -> (w400:ext)
                        n170 = local read "Chirp start (MHz)"() -> (w399:ext)
                        n171 = local read "Ampl. (dBm)"() -> (w398:dbl)
                        n172 = local read "f start (MHz)"() -> (w395:dbl)
                        n173 = local read "f step (MHz)"() -> (w394:dbl)
                        n174 = local read "#steps"() -> (w393:u32)
                        n175 = call "t2point.vi"("t/point"=w404) -> ("ps/point"=w396:u32)
                        n176 = call "t2ns.vi"("t/div"=w403) -> ("ns/div"=w397:u32)
                        n177 = local read "Folder"() -> (w389:path)
                        n178 = local read "Name"() -> (w388:string)
                        n179 = local read "Ext"() -> (w385:string)
                        n180 = Path To String(path=w389) -> (string=w392:string)
                        n181 = Format Into String(format string="Channel: %d\\nps/point: %d\\nns/div: %d\\nAmount of averagings: %d\\n#Sweeps: %d\\nFilter up to (MHz): %f\\nChirp start (MHz): %f\\nAmpl. (dBm): %f\\nf start (MHz): %f\\nf step (MHz): %f\\n#steps: %d\\n", w405, w396, w397, w402, w401, w400, w399, w398, w395, w394, w393) -> (resulting string=w376:string)  [unwired: 2 in, 1 out]
                        n182 = Concatenate Strings(w392, "\\\\" ("string"), w388, "_", "par", ".", w385) -> (w384:string)
                        n183 = case shown="False" w375 {
                          tunnel: [T3."replace or create with confirmation" ("operation (0:open)") T3."replace or create" ("operation (0:open)")] -> w374
                          frame #0 {
                          }
                          frame #1 {
                          }
                        }
                        n184 = String To Path(string=w384) -> (path=w378:path)
                        n185 = Open/Create/Replace File(file path (use dialog)=w378, operation (0:open)=w374, access (0:read/write)=enum16{"read/write", "read-only", "write-only"}."write-only") -> (refnum out=w380:refnum<file>, error out=w383:errorcluster)  [unwired: 3 in, 1 out]
                        n186 = Write to Text File(file (use dialog)=w380, text=w376, error in=w383) -> (refnum out=w381:refnum<file>, error out=w382:errorcluster)  [unwired: 1 in, 1 out]
                        n187 = Close File(refnum=w381, error in=w382) -> (error out=w379:errorcluster)  [unwired: 1 out]
                        n188 = call <vilib>:"Simple Error Handler.vi"("error in (no error)"=w379) -> ()  [unwired: 4 in, 5 out]
                      }
                    }
                    n189 = local write "Stop"(FALSE ("Stop")) -> ()
                  }
                }
              }
            }
          }
        }
        n190 = Wait Until Next ms Multiple(millisecond multiple=u32 150) -> ()  [unwired: 1 out]
      }
    }
    frame #2 {
      n191 = Current VI's Path() -> (path=w417:path)
      n192 = Strip Path(path=w417) -> (stripped path=w418:path)  [unwired: 1 out]
      n193 = Build Path(base path=w418, name or relative path="Data_get.cfg") -> (appended path=w420:path)
      n194 = call "SaveControlValues.vi"("file path"=w420, "vi path"=w417) -> ("error out"=w419:errorcluster)
      n195 = call <vilib>:"Simple Error Handler.vi"("error in (no error)"=w419) -> ()  [unwired: 4 in, 5 out]
    }
  }
